vi "Send Message.vi"(7 "message":string, 8 "error in (no error)":errorcluster, 9 "slack channel":string, 10 "slack API token":string) -> (0 "error out":errorcluster, 1 "slack channel dup":string, 2 "slack API token dup":string)   [LabVIEW 2019, in "Slack API.lvlib"]
uses:
  Slack API.lvlib
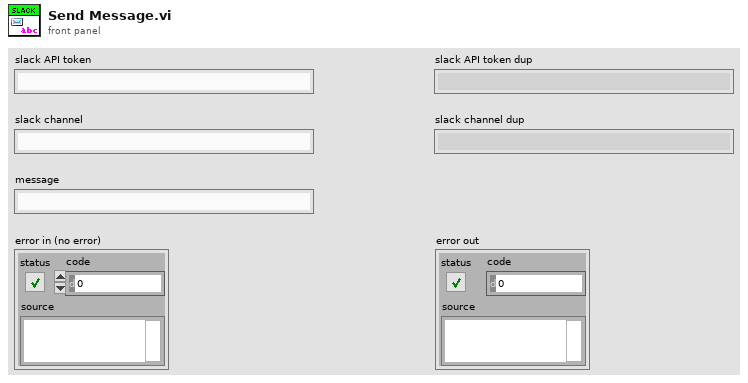
[diagram p1: front panel]
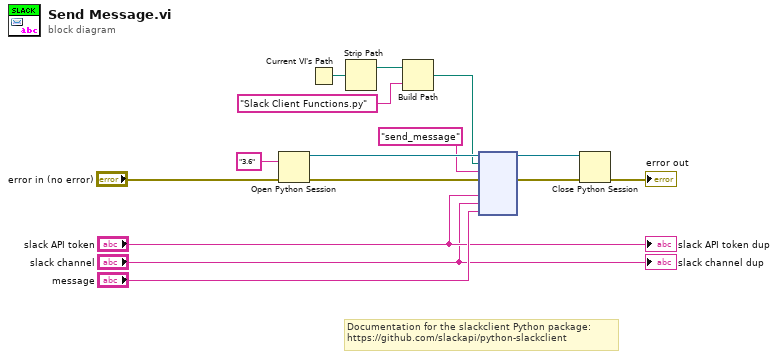
[diagram p0: block diagram]
diagram:
  # "Documentation for the slackclient Python package:\nhttps://github.com/slackapi/python-slackclient"
  n1 = Open Python Session(python version="3.6" ("Python version"), 3:"error in (no error)") -> (session out=w14:refnum<k35>, error out=w12:errorcluster)  [unwired: 1 in]
  n2 = Current VI's Path() -> (path=w8:path)
  n3 = Strip Path(path=w8) -> (stripped path=w7:path)  [unwired: 1 out]
  n4 = Build Path(base path=w7, name or relative path="Slack Client Functions.py") -> (appended path=w6:path)
  n5 = node(w14, w6, "send_message" ("function name"), w12, "slack API token", "slack channel", "message") -> (w9:refnum<k35>, w10:errorcluster)  [unwired: 5 in, 2 out]
  n6 = Close Python Session(session in=w9, error in=w10) -> (11:→"error out":errorcluster)
  "slack API token dup" <- "slack API token"
  "slack channel dup" <- "slack channel"
